vi "Init.vi"(8 "error in (no error)":errorcluster, 11 "Configuration Window in":refnum<class "Configuration Window.lvclass">) -> (0 "error out":errorcluster, 3 "Configuration Window out":refnum<class "Configuration Window.lvclass">)   [LabVIEW 2018, in "Configuration Window.lvlib" / "Configuration Window.lvclass"]
uses:
  Configuration Window.lvclass
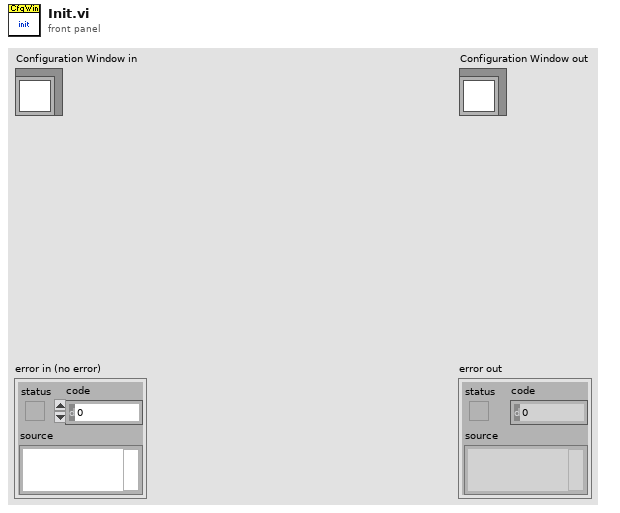
[diagram p1: front panel]
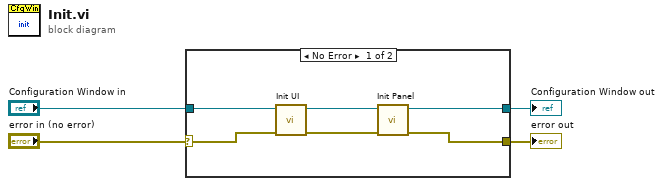
[diagram p0: block diagram]
diagram:
  n1 = case shown="No Error" "error in (no error)" {
    selector: "error in (no error)" -> [w5 w12]
    tunnel: [w6 w12] -> w3
    tunnel: [w7 w11] -> w1
    tunnel: "Configuration Window in" -> [w8 w11]
    frame No Error {
      n2 = call "Init UI.vi"("error in (no error)"=w5, "Configuration Window in"=w8) -> ("error out"=w9:errorcluster, "Configuration Window out"=w10:refnum<class "Configuration Window.lvclass">)  [unwired: 8 in]
      n3 = call "Init Panel.vi"("error in (no error)"=w9, "Configuration Window in"=w10) -> ("error out"=w6:errorcluster, "Configuration Window out"=w7:refnum<class "Configuration Window.lvclass">)  [unwired: 8 in]
    }
    frame Error {
    }
  }
  "error out" <- w3
  "Configuration Window out" <- w1
